vi "blink.vi"() -> ()   [LabVIEW 2015]
uses:
  global.vi
panel:
  out "Numeric":dbl
  out "Boolean":bool
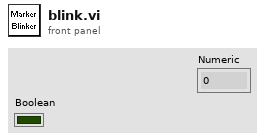
[diagram p1: front panel]
types:
  T1 = cluster{"Airspeed":dbl, "Altitude":dbl, "Vertical Speed":dbl, "Pitch":dbl, "Roll":dbl, "Heading":dbl, "Turn Indicator":dbl, "Latitude":dbl, "Longitude":dbl, "pilot g":dbl, "view number":i16, "fov":dbl, "view heading":dbl, "view pitch":dbl, "game width":i16, "game height":i16}
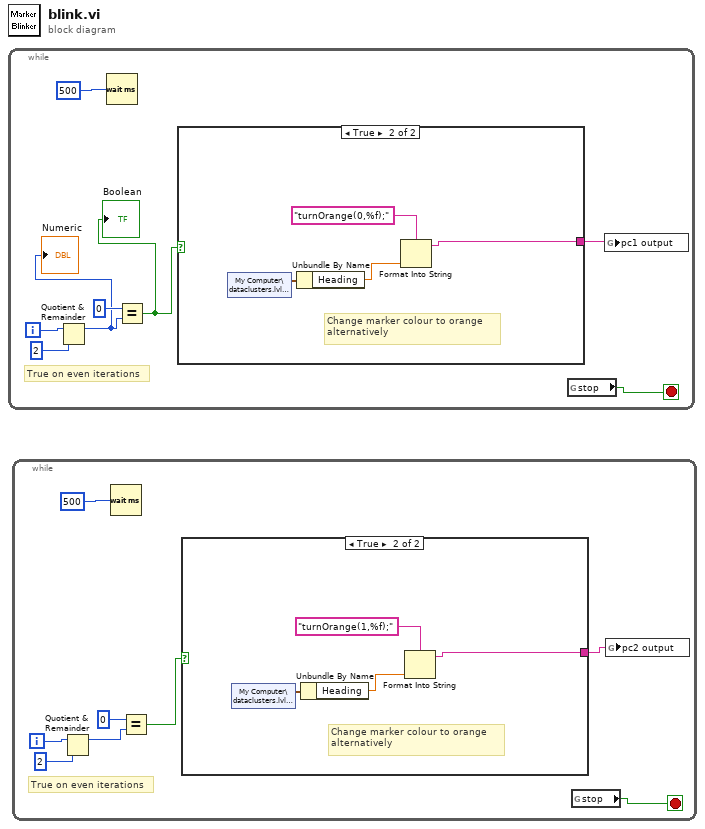
[diagram p0: block diagram]
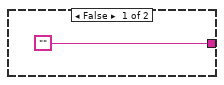
[diagram p2: hidden frame]
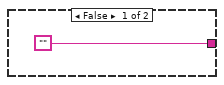
[diagram p3: hidden frame]
diagram:
  n1 = while {
    i -> [w7]
    stop <- w4 stop-if-true
    # "True on even iterations"
    n2 = Quotient & Remainder(x=w7, y=2) -> (x-y*floor(x/y)=w1:i32)  [unwired: 1 out]
    "Numeric" <- w1
    n3 = Wait (ms)(milliseconds to wait=u32 500) -> ()  [unwired: 1 out]
    n4 = Equal?(x=0, y=w1) -> (x = y?=w2:bool)
    "Boolean" <- w2
    n5 = case shown="True" w2 {
      tunnel: ["" w10] -> w3
      frame False {
      }
      frame True {
        # "Change marker colour to orange\nalternatively"
        n6 = shared-variable "My Computer\\dataclusters.lvlib\\pc1"() -> (w12:T1)  [unwired: 1 in, 1 out]
        n7 = Unbundle By Name(w12) -> ("Heading"=w11:dbl)
        n8 = Format Into String(format string="turnOrange(0,%f);", w11) -> (resulting string=w10:string)  [unwired: 2 in, 1 out]
      }
    }
    n9 = global read "global.vi" "stop"() -> (w4:bool)
    n10 = global write "global.vi" "pc1 output"(w3) -> ()
  }
  n11 = while {
    i -> [w20]
    stop <- w15 stop-if-true
    # "True on even iterations"
    n12 = Quotient & Remainder(x=w20, y=2) -> (x-y*floor(x/y)=w18:i32)  [unwired: 1 out]
    n13 = Wait (ms)(milliseconds to wait=u32 500) -> ()  [unwired: 1 out]
    n14 = Equal?(x=0, y=w18) -> (x = y?=w16:bool)
    n15 = case shown="True" w16 {
      tunnel: ["" w23] -> w14
      frame False {
      }
      frame True {
        # "Change marker colour to orange\nalternatively"
        n16 = shared-variable "My Computer\\dataclusters.lvlib\\pc2"() -> (w25:T1)  [unwired: 1 in, 1 out]
        n17 = Unbundle By Name(w25) -> ("Heading"=w24:dbl)
        n18 = Format Into String(format string="turnOrange(1,%f);", w24) -> (resulting string=w23:string)  [unwired: 2 in, 1 out]
      }
    }
    n19 = global read "global.vi" "stop"() -> (w15:bool)
    n20 = global write "global.vi" "pc2 output"(w14) -> ()
  }
